vi "addCategory.vi"(8 "Error In":errorcluster, 10 "category":refnum<class "QWinJumpListCategory.lvclass">, 11 "QWinJumpList In":refnum<class "QWinJumpList.lvclass">) -> (0 "Error Out":errorcluster, 3 "QWinJumpList Out":refnum<class "QWinJumpList.lvclass">)   [LabVIEW 2014, in "QWinJumpList.lvclass"]
doc: "LabVIEW-specific documentation is not yet available."
uses:
  QWinJumpList.lvclass
  QWinJumpListCategory/QWinJumpListCategory.lvclass
  LQ Core/LQIdentity/LQIdentity.lvclass/LQIdentity.ctl
  LQ Core/LQ Core.lvlib
  LQ Core/LQIdentity/LQIdentity.lvclass
panel:
  # "Copyright (c) 2016 Sze Howe Koh\n\nThis Source Code Form is subject to the terms of the Mozilla Public\nLicense, v. 2.0. If a copy of the MPL was not distributed with this\nfile, You can obtain one at http://mozilla.org/MPL/2.0/."
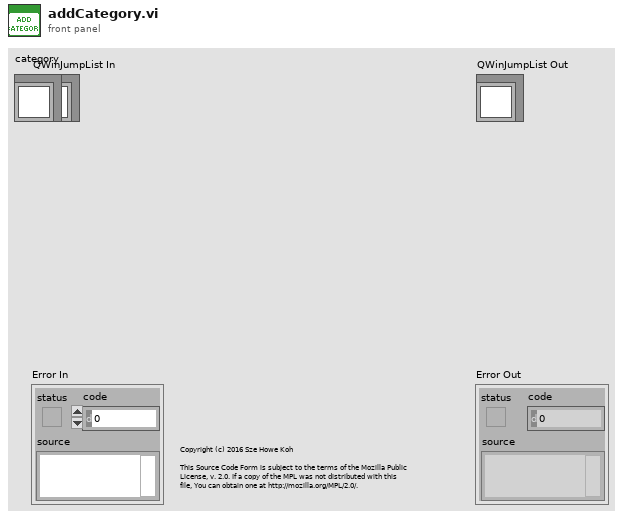
[diagram p1: front panel]
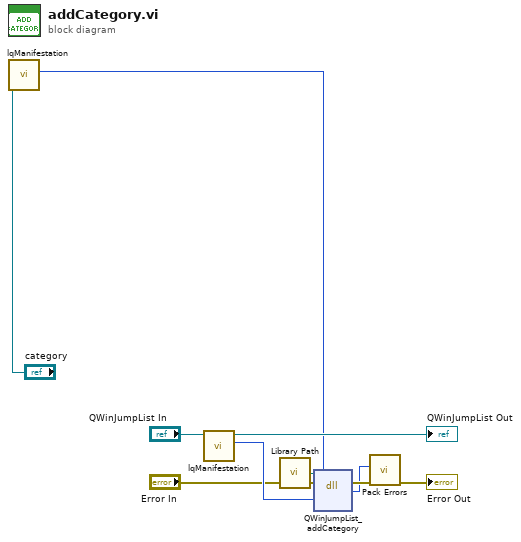
[diagram p0: block diagram]
diagram:
  n1 = call "lqManifestation.vi"("LQIdentity in"="category") -> ("Manifestation"=w1:u64)  [unwired: 9 in, 1 out]
  n2 = call "lqManifestation.vi"("LQIdentity in"="QWinJumpList In") -> ("Manifestation"=w7:u64, "LQIdentity out"=→"QWinJumpList Out":refnum<class "QWinJumpList.lvclass">)  [unwired: 9 in]
  n3 = call "Library Path.vi"() -> ("Library Path"=w8:path)
  n4 = dll-call lib="?" fn="QWinJumpList_addCategory"(path in=w8, error in="Error In", "_instance"=w7, "category"=w1) -> (error out=w5:errorcluster, w3:i32)  [unwired: 3 in, 1 out]
  n5 = call "Pack Errors.vi"("Error In"=w5, "Error Code"=w3) -> ("Error Out"=→"Error Out":errorcluster)  [unwired: 9 in]
